vi "Append unique suffix.vi"(6 "Extention":string, 7 "Suffix":string, 8 "error in (no error)":errorcluster, 11 "Path":path) -> (0 "error out":errorcluster, 3 "Path out":path)   [LabVIEW 2015]
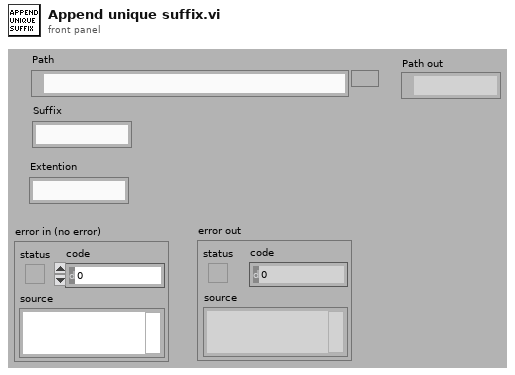
[diagram p1: front panel]
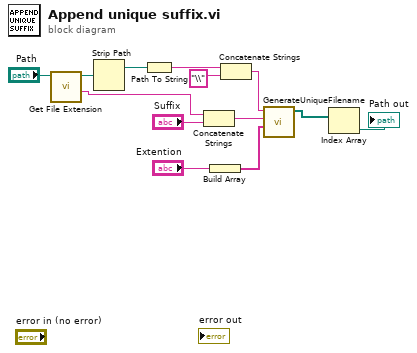
[diagram p0: block diagram]
diagram:
  n1 = call <vilib>:"Get File Extension.vi"("file"="Path") -> ("filename without extension"=w6:string, "dup file"=w5:path)  [unwired: 6 in, 3 out]
  n2 = Strip Path(path=w5) -> (stripped path=w9:path)  [unwired: 1 out]
  n3 = Path To String(path=w9) -> (string=w8:string)
  n4 = Concatenate Strings(w6, "Suffix") -> (w12:string)
  n5 = Build Array("Extention") -> (w10:string[])
  n6 = Concatenate Strings(w8, "\\" ("string")) -> (w4:string)
  n7 = call "GenerateUniqueFilename.vi"("File Name Suffixes"=w10, "File Name Prefix"=w12, "Folder"=w4) -> ("Paths"=w2:path[])  [unwired: 7 in, 1 out]
  n8 = Index Array(array=w2) -> (element=→"Path out":path)  [unwired: 1 in]
